vi "Configure Normal Dimmer Mode.vi"(8 "error in":errorcluster, 10 "Mode":u16(ring) items=["OFF", "Leading", "Trailing"], 11 "VISA resource name":refnum<visa-resource-name>) -> (0 "error out":errorcluster, 3 "VISA resource name out":refnum<visa-resource-name>)   [LabVIEW 2020, in "IT-M7700.lvlib"]
doc: "This command is used to set the phase dimming mode.\n<b>Mode</b>\n0: OFF\n1: Leading\n2: Trailing"
uses:
  <instrlib>/IT-M7700/IT-M7700.lvlib
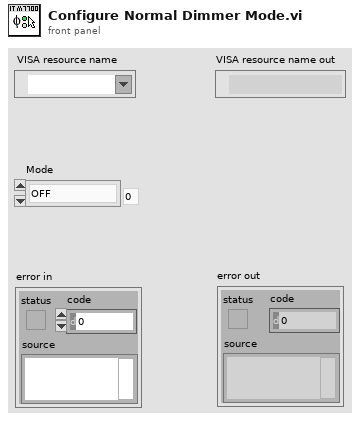
[diagram p1: front panel]
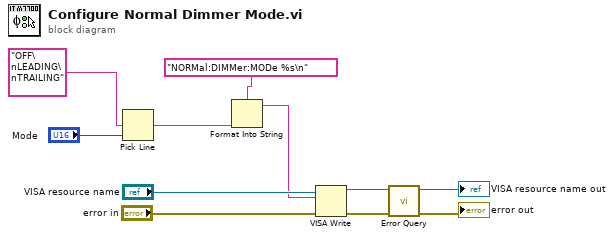
[diagram p0: block diagram]
diagram:
  n1 = Pick Line(multi-line string="OFF\nLEADING\nTRAILING", line index="Mode") -> (output string=w1:string)  [unwired: 1 in]
  n2 = Format Into String(format string="NORMal:DIMMer:MODe %s\n", w1) -> (resulting string=w8:string)  [unwired: 2 in, 1 out]
  n3 = VISA Write(VISA resource name="VISA resource name", write buffer=w8, error in (no error)="error in") -> (VISA resource name out=w7:refnum<visa-resource-name>, error out=w6:errorcluster)  [unwired: 1 out]
  n4 = call <instrlib>:"Error Query.vi"("error in"=w6, "VISA resource name"=w7) -> ("error out"=→"error out":errorcluster, "VISA resource name out"=→"VISA resource name out":refnum<visa-resource-name>)  [unwired: 6 in, 2 out]
